vi "Get Master Scan Enable.vi"(8 "error in (no error)":errorcluster, 11 "hdl in":i32) -> (0 "error out":errorcluster, 2 "Master Scan Enable?":bool, 3 "hdl out":i32)   [LabVIEW 2011, in "Thorlabs_MDT69xB.lvlib"]
doc: "Returns the state of the Master Scan enable."
uses:
  <instrlib>/Thorlabs_MDT69xB/Thorlabs_MDT69xB.lvlib
  <instrlib>/Thorlabs_MDT69xB/Data/MDT_COMMAND_LIB_win32.dll
  <instrlib>/Thorlabs_MDT69xB/Data/MDT_COMMAND_LIB_x64.dll
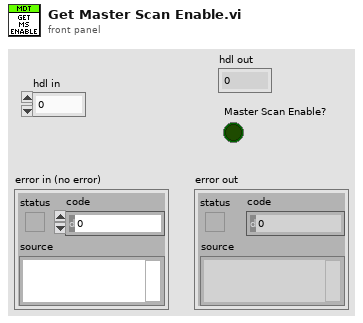
[diagram p1: front panel]
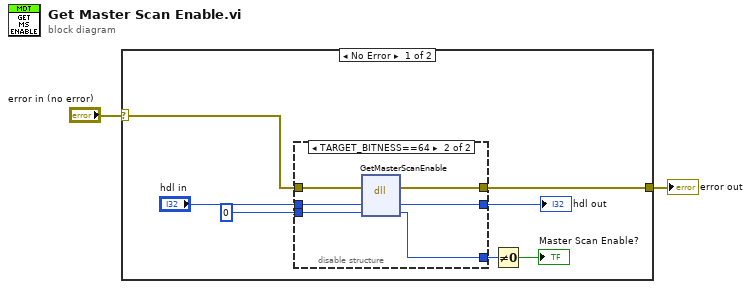
[diagram p0: block diagram]
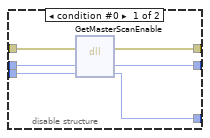
[diagram p2: hidden frame]
diagram:
  n1 = case shown="No Error" "error in (no error)" {
    selector: "error in (no error)" -> [w9 w22]
    tunnel: [w6 w22] -> w1
    frame No Error {
      n2 = disable-structure shown="TARGET_BITNESS==64" {
        disable-tunnel: w9 -> [w15 w21]
        disable-tunnel: "hdl in" -> [w14 w20]
        disable-tunnel: 0 ("State") -> [w13 w19]
        disable-tunnel: [w12 w18] -> w6
        disable-tunnel: [w11 w17] -> w4
        disable-tunnel: [w10 w16] -> w3
        frame condition #0 {
          n3 = dll-call lib="E:/Program Files (x86)/National Instruments/LabVIEW 2011/instr.lib/Thorlabs_MDT69xB/Data/MDT_COMMAND_LIB_win32.dll" fn="GetMasterScanEnable"(error in=w15, "hdl"=w14, "State"=w13) -> (error out=w12:errorcluster, "hdl"=w10:i32, "State"=w11:i32)  [unwired: 3 in, 1 out]
        }
        frame condition #1 (active) {
          n4 = dll-call lib="C:/Program Files/National Instruments/LabVIEW 2011/instr.lib/Thorlabs_MDT69xB/Data/MDT_COMMAND_LIB_x64.dll" fn="GetMasterScanEnable"(error in=w21, "hdl"=w20, "State"=w19) -> (error out=w18:errorcluster, "hdl"=w16:i32, "State"=w17:i32)  [unwired: 3 in, 1 out]
        }
      }
      "hdl out" <- w3
      n5 = Not Equal To 0?(x=w4) -> (x != 0?=→"Master Scan Enable?":bool)
    }
    frame Error {
    }
  }
  "error out" <- w1
